vi "JTAG Base Function.vi"(0 "Function":u16(ring) items=["READ_IO_VARS"=0, "PORT_OUT"=1, "PORT_SEL"=2, "PORT_REN"=3, "PORT_IN"=4, "PORT_DIR"=5, "SET_LCM"=6, "PWR_WRITE_SINGLE"=12, "PWR_READ_SINGLE"=13, "PWR_WRITE_MASK"=16, "PWR_WRITE_TRIM_DEFAULTS"=17, "STIM_POWER_UP"=20, "STIM_POWER_DN"=21, "STIM_WRITE_SINGLE"=22, "STIM_READ_SINGLE"=23, "STIM_WRITE_BLOCK"=24, "STIM_READ_BLOCK"=25, "STIM_WRITE_MASK"=26, "MICS_POWER_UP"=30, "MICS_WAKEUP_PULSE"=205, "MICS_POWER_DN"=31, "MICS_WRITE_SINGLE"=32, "MICS_READ_SINGLE"=33, "MICS_WRITE_BLOCK"=34, "MICS_READ_BLOCK"=35, "MICS_WRITE_MASK"=36, "MEM_POWER_UP"=40, "MEM_POWER_DN"=41, "MEM_WRITE_SINGLE"=42, "MEM_READ_SINGLE"=43, "MEM_WRITE_BLOCK"=44, "MEM_READ_BLOCK"=45, "MEM_WRITE_MASK"=46, "MEM_WRITE_SR"=47, "MEM_READ_SR"=48, "MEM_WRITE_OPCODE"=49, "INIT_PORTS"=50, "INIT_COMMS"=60, "RELEASE_COMMS"=61, "INIT_VARS"=62, "DCO_1MHZ"=63, "DCO_8MHZ"=64, "STANDARD_STARTUP"=65, "SET_LCM"=66, "PLUTO_WRITE_TRIM_DEFAULTS"=67, "SATURN_DIG_STARTUP"=68, "SATURN_BBC_STARTUP"=69, "SATURN_BBC_SHUTDOWN"=70, "SATURN_AUTO_FULL_STARTUP"=71, "SATURN_FULL_SHUTDOWN"=72, "SATURN_ENABLE_PROGRAMMING"=73, "SATURN_ENABLE_SEQUENCER"=74, "START_STIM_CLK"=80, "STOP_STIM_CLK"=81, "PULSE_STIM_CLK"=82, "PULSE_STIM_SCK"=83, "SINGLE_ADC12"=85, "SINGLE_ADC12_REPEAT"=86, "MULTI_ADC12"=87, "MULTI_ADC12_REPEAT"=88, "DISABLE_ADC12"=89, "READ_CLOCK_REGISTERS"=90, "WRITE_CLOCK_REGISTERS"=91, "TC_STIM_RAM_READ"=200, "TC_STIM_RAM_WRITE"=201, "TC_STIM_PHASE_REGS_READ"=202, "TC_STIM_PHASE_REGS_WRITE"=203, "TC_BROWN_OUT_TEST"=204, "TC_TIMING_TEST"=220], 1 "ARG 4":u16 format="%04x", 2 "ARG 5":u16 format="%04x", 3 "ARG 6":u16 format="%04x", 5 "ARG 1":u16 format="%04x", 7 "ARG 2":u16 format="%04x", 9 "ARG 3":u16 format="%04x", 11 "error in (no error)":errorcluster) -> (4 "ARG 7":u16 format="%04x", 8 "ARG1-ARG7":u16[](array[numeric]) format="%04x", 15 "error out":errorcluster)   [LabVIEW 2010]
panel:
  # "ARG1"
  # "ARG2"
  # "ARG3"
  # "ARG4"
  # "ARG5"
  # "ARG6"
  # "ARG7"
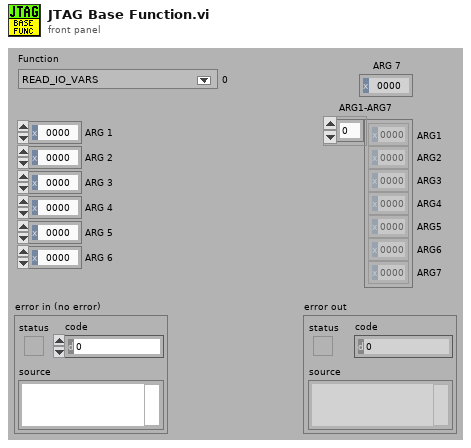
[diagram p1: front panel]
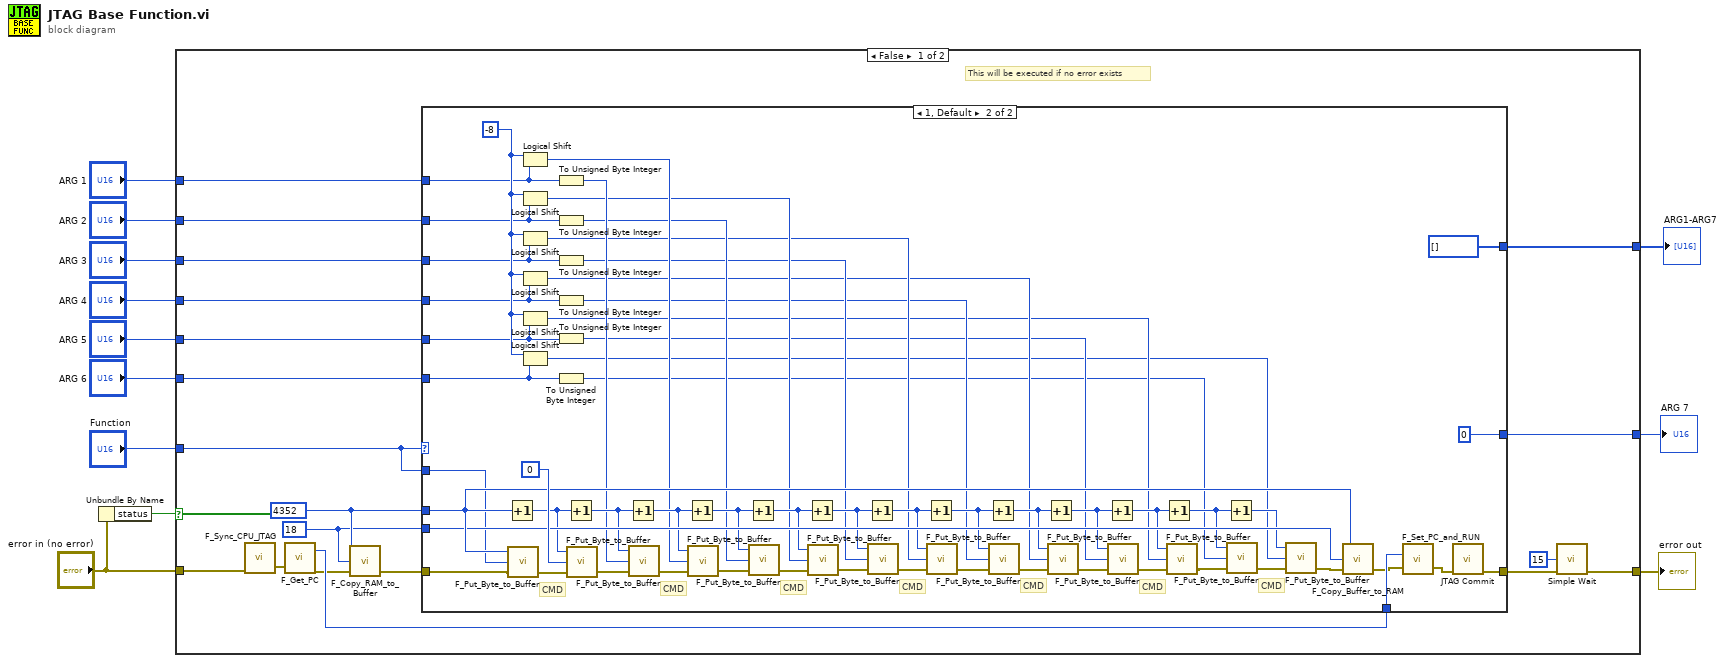
[diagram p0: block diagram]
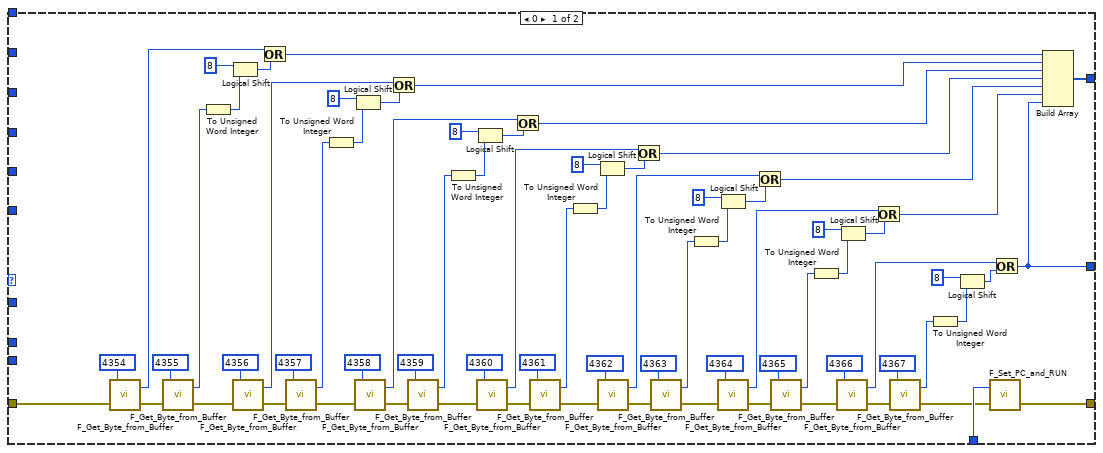
[diagram p2: hidden frame]
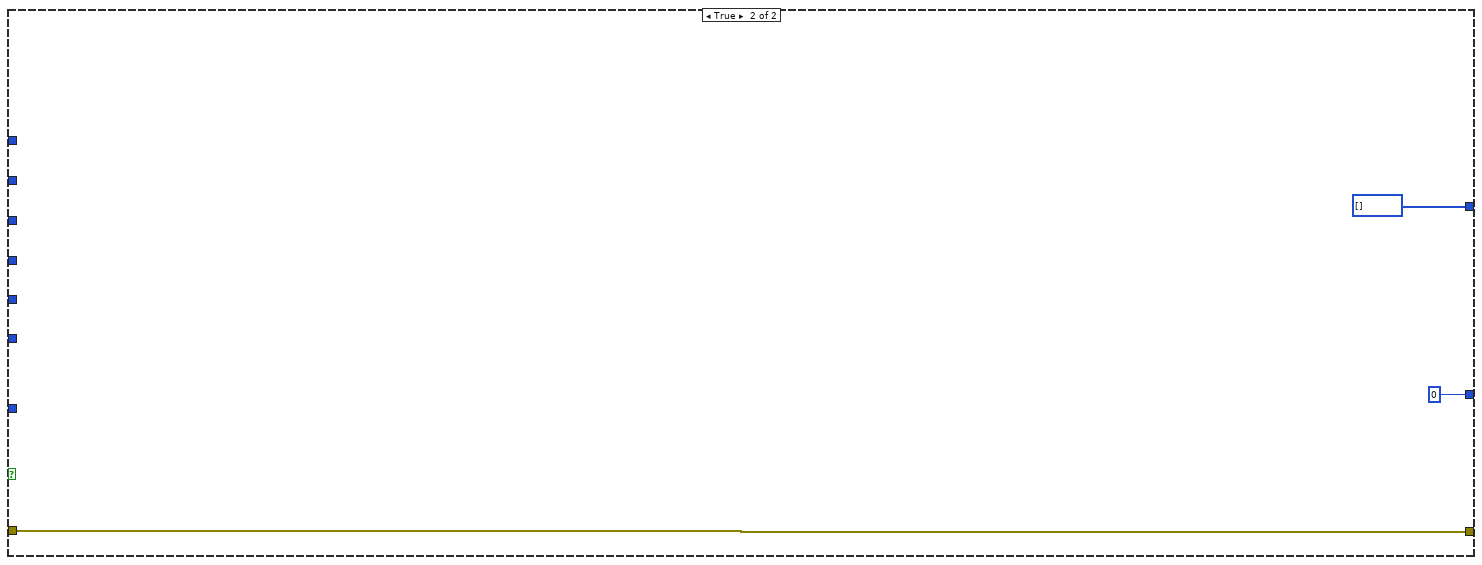
[diagram p3: hidden frame]
diagram:
  n1 = Unbundle By Name("error in (no error)") -> ("status"=w11:bool)
  n2 = case shown="False" w11 {
    tunnel: [w16 w165] -> w12
    tunnel: "error in (no error)" -> [w31 w165]
    tunnel: "Function" -> [w13 _]
    tunnel: "ARG 6" -> [w20 _]
    tunnel: "ARG 5" -> [w21 _]
    tunnel: "ARG 4" -> [w22 _]
    tunnel: "ARG 3" -> [w23 _]
    tunnel: "ARG 2" -> [w24 _]
    tunnel: "ARG 1" -> [w25 _]
    tunnel: [w15 u16 0 ("ARG 7")] -> w3
    tunnel: [w14 u16[] []] -> w2
    frame False {
      w29 = u16 18
      w30 = u16 4352
      # "This will be executed if no error exists"
      n3 = call "F_Sync_CPU_JTAG.vi"("error in (no error)"=w31) -> ("error out"=w27:errorcluster)  [unwired: 1 in, 1 out]
      n4 = call "F_Get_PC.vi"("error in (no error)"=w27) -> ("error out"=w19:errorcluster, "Program Counter"=w26:u16)  [unwired: 1 in]
      n5 = call "F_Copy_RAM_to_Buffer.vi"("error in (no error)"=w19, "Block size to be copied"=w29, "RAM start address"=w30) -> ("error out"=w28:errorcluster)  [unwired: 2 in]
      n6 = case shown="1, Default" w13 {
        tunnel: w30 -> [_ w160]
        tunnel: w29 -> [_ w159]
        tunnel: w28 -> [w58 w158]
        tunnel: w13 -> [_ w157]
        tunnel: w26 -> [w105 w156]
        tunnel: w25 -> [_ w128]
        tunnel: w24 -> [_ w127]
        tunnel: w23 -> [_ w126]
        tunnel: w22 -> [_ w125]
        tunnel: w21 -> [_ w124]
        tunnel: w20 -> [_ w123]
        tunnel: [w104 w108] -> w17
        tunnel: [w51 u16 0 ("ARG 7")] -> w15
        tunnel: [w32 u16[] []] -> w14
        frame 0 {
          n7 = call "F_Get_Byte_from_Buffer.vi"("error in (no error)"=w58, "Address of byte to be read"=u16 4354) -> ("error out"=w64:errorcluster, "Current value"=w44:u8)
          n8 = call "F_Get_Byte_from_Buffer.vi"("error in (no error)"=w64, "Address of byte to be read"=u16 4355) -> ("error out"=w52:errorcluster, "Current value"=w60:u8)
          n9 = To Unsigned Word Integer(number=w60) -> (unsigned 16bit integer=w59:u16)
          n10 = Logical Shift(y=i16 8, x=w59) -> (x << y=w50:u16)
          n11 = call "F_Get_Byte_from_Buffer.vi"("error in (no error)"=w52, "Address of byte to be read"=u16 4356) -> ("error out"=w70:errorcluster, "Current value"=w43:u8)
          n12 = Or(x=w44, y=w50) -> (x .or. y?=w33:u16)
          n13 = call "F_Get_Byte_from_Buffer.vi"("error in (no error)"=w70, "Address of byte to be read"=u16 4357) -> ("error out"=w53:errorcluster, "Current value"=w66:u8)
          n14 = To Unsigned Word Integer(number=w66) -> (unsigned 16bit integer=w65:u16)
          n15 = Logical Shift(y=i16 8, x=w65) -> (x << y=w49:u16)
          n16 = call "F_Get_Byte_from_Buffer.vi"("error in (no error)"=w53, "Address of byte to be read"=u16 4358) -> ("error out"=w76:errorcluster, "Current value"=w42:u8)
          n17 = Or(x=w43, y=w49) -> (x .or. y?=w34:u16)
          n18 = call "F_Get_Byte_from_Buffer.vi"("error in (no error)"=w76, "Address of byte to be read"=u16 4359) -> ("error out"=w54:errorcluster, "Current value"=w72:u8)
          n19 = To Unsigned Word Integer(number=w72) -> (unsigned 16bit integer=w71:u16)
          n20 = Logical Shift(y=i16 8, x=w71) -> (x << y=w48:u16)
          n21 = call "F_Get_Byte_from_Buffer.vi"("error in (no error)"=w54, "Address of byte to be read"=u16 4360) -> ("error out"=w82:errorcluster, "Current value"=w41:u8)
          n22 = Or(x=w42, y=w48) -> (x .or. y?=w35:u16)
          n23 = call "F_Get_Byte_from_Buffer.vi"("error in (no error)"=w82, "Address of byte to be read"=u16 4361) -> ("error out"=w55:errorcluster, "Current value"=w78:u8)
          n24 = To Unsigned Word Integer(number=w78) -> (unsigned 16bit integer=w77:u16)
          n25 = Logical Shift(y=i16 8, x=w77) -> (x << y=w47:u16)
          n26 = call "F_Get_Byte_from_Buffer.vi"("error in (no error)"=w55, "Address of byte to be read"=u16 4362) -> ("error out"=w88:errorcluster, "Current value"=w40:u8)
          n27 = Or(x=w41, y=w47) -> (x .or. y?=w36:u16)
          n28 = call "F_Get_Byte_from_Buffer.vi"("error in (no error)"=w88, "Address of byte to be read"=u16 4363) -> ("error out"=w56:errorcluster, "Current value"=w84:u8)
          n29 = To Unsigned Word Integer(number=w84) -> (unsigned 16bit integer=w83:u16)
          n30 = Logical Shift(y=i16 8, x=w83) -> (x << y=w46:u16)
          n31 = call "F_Get_Byte_from_Buffer.vi"("error in (no error)"=w56, "Address of byte to be read"=u16 4364) -> ("error out"=w94:errorcluster, "Current value"=w39:u8)
          n32 = Or(x=w40, y=w46) -> (x .or. y?=w37:u16)
          n33 = call "F_Get_Byte_from_Buffer.vi"("error in (no error)"=w94, "Address of byte to be read"=u16 4365) -> ("error out"=w57:errorcluster, "Current value"=w90:u8)
          n34 = To Unsigned Word Integer(number=w90) -> (unsigned 16bit integer=w89:u16)
          n35 = call "F_Get_Byte_from_Buffer.vi"("error in (no error)"=w57, "Address of byte to be read"=u16 4366) -> ("error out"=w103:errorcluster, "Current value"=w99:u8)
          n36 = Logical Shift(y=i16 8, x=w89) -> (x << y=w45:u16)
          n37 = Or(x=w39, y=w45) -> (x .or. y?=w38:u16)
          n38 = call "F_Get_Byte_from_Buffer.vi"("error in (no error)"=w103, "Address of byte to be read"=u16 4367) -> ("error out"=w102:errorcluster, "Current value"=w96:u8)
          n39 = To Unsigned Word Integer(number=w96) -> (unsigned 16bit integer=w95:u16)
          n40 = Logical Shift(y=i16 8, x=w95) -> (x << y=w97:u16)
          n41 = call "F_Set_PC_and_RUN.vi"("error in (no error)"=w102, "PC start address"=w105) -> ("error out"=w104:errorcluster)  [unwired: 1 in]
          n42 = Or(x=w99, y=w97) -> (x .or. y?=w51:u16)
          n43 = Build Array(w33, w34, w35, w36, w37, w38, w51) -> (w32:u16[])
        }
        frame 1, Default {
          w130 = -8
          # "CMD"
          # "CMD"
          # "CMD"
          # "CMD"
          # "CMD"
          # "CMD"
          # "CMD"
          n44 = Increment(x=w160) -> (x+1=w148:u16)
          n45 = call "F_Put_Byte_to_Buffer.vi"("error in (no error)"=w158, "New value"=w157, "Address of byte to be updated"=w160) -> ("error out"=w162:errorcluster)  [unwired: 2 in]
          n46 = Logical Shift(y=w130, x=w128) -> (x << y=w129:u16)
          n47 = Logical Shift(y=w130, x=w127) -> (x << y=w120:u16)
          n48 = Logical Shift(y=w130, x=w126) -> (x << y=w118:u16)
          n49 = Logical Shift(y=w130, x=w125) -> (x << y=w116:u16)
          n50 = Logical Shift(y=w130, x=w124) -> (x << y=w114:u16)
          n51 = Logical Shift(y=w130, x=w123) -> (x << y=w113:u16)
          n52 = To Unsigned Byte Integer(number=w128) -> (unsigned 8bit integer=w122:u8)
          n53 = To Unsigned Byte Integer(number=w127) -> (unsigned 8bit integer=w121:u8)
          n54 = To Unsigned Byte Integer(number=w126) -> (unsigned 8bit integer=w119:u8)
          n55 = To Unsigned Byte Integer(number=w125) -> (unsigned 8bit integer=w117:u8)
          n56 = To Unsigned Byte Integer(number=w124) -> (unsigned 8bit integer=w115:u8)
          n57 = To Unsigned Byte Integer(number=w123) -> (unsigned 8bit integer=w112:u8)
          n58 = Increment(x=w148) -> (x+1=w147:u16)
          n59 = call "F_Put_Byte_to_Buffer.vi"("error in (no error)"=w162, "New value"=u16 0, "Address of byte to be updated"=w148) -> ("error out"=w131:errorcluster)  [unwired: 2 in]
          n60 = Increment(x=w147) -> (x+1=w146:u16)
          n61 = call "F_Put_Byte_to_Buffer.vi"("error in (no error)"=w131, "New value"=w122, "Address of byte to be updated"=w147) -> ("error out"=w155:errorcluster)  [unwired: 2 in]
          n62 = Increment(x=w146) -> (x+1=w145:u16)
          n63 = call "F_Put_Byte_to_Buffer.vi"("error in (no error)"=w155, "New value"=w129, "Address of byte to be updated"=w146) -> ("error out"=w132:errorcluster)  [unwired: 2 in]
          n64 = Increment(x=w145) -> (x+1=w144:u16)
          n65 = call "F_Put_Byte_to_Buffer.vi"("error in (no error)"=w132, "New value"=w121, "Address of byte to be updated"=w145) -> ("error out"=w154:errorcluster)  [unwired: 2 in]
          n66 = Increment(x=w144) -> (x+1=w143:u16)
          n67 = call "F_Put_Byte_to_Buffer.vi"("error in (no error)"=w154, "New value"=w120, "Address of byte to be updated"=w144) -> ("error out"=w133:errorcluster)  [unwired: 2 in]
          n68 = Increment(x=w143) -> (x+1=w142:u16)
          n69 = call "F_Put_Byte_to_Buffer.vi"("error in (no error)"=w133, "New value"=w119, "Address of byte to be updated"=w143) -> ("error out"=w153:errorcluster)  [unwired: 2 in]
          n70 = Increment(x=w142) -> (x+1=w141:u16)
          n71 = call "F_Put_Byte_to_Buffer.vi"("error in (no error)"=w153, "New value"=w118, "Address of byte to be updated"=w142) -> ("error out"=w134:errorcluster)  [unwired: 2 in]
          n72 = Increment(x=w141) -> (x+1=w140:u16)
          n73 = call "F_Put_Byte_to_Buffer.vi"("error in (no error)"=w134, "New value"=w117, "Address of byte to be updated"=w141) -> ("error out"=w152:errorcluster)  [unwired: 2 in]
          n74 = Increment(x=w140) -> (x+1=w139:u16)
          n75 = call "F_Put_Byte_to_Buffer.vi"("error in (no error)"=w152, "New value"=w116, "Address of byte to be updated"=w140) -> ("error out"=w135:errorcluster)  [unwired: 2 in]
          n76 = Increment(x=w139) -> (x+1=w138:u16)
          n77 = call "F_Put_Byte_to_Buffer.vi"("error in (no error)"=w135, "New value"=w115, "Address of byte to be updated"=w139) -> ("error out"=w151:errorcluster)  [unwired: 2 in]
          n78 = Increment(x=w138) -> (x+1=w137:u16)
          n79 = call "F_Put_Byte_to_Buffer.vi"("error in (no error)"=w151, "New value"=w114, "Address of byte to be updated"=w138) -> ("error out"=w136:errorcluster)  [unwired: 2 in]
          n80 = Increment(x=w137) -> (x+1=w149:u16)
          n81 = call "F_Put_Byte_to_Buffer.vi"("error in (no error)"=w136, "New value"=w112, "Address of byte to be updated"=w137) -> ("error out"=w150:errorcluster)  [unwired: 2 in]
          n82 = call "F_Put_Byte_to_Buffer.vi"("error in (no error)"=w150, "New value"=w113, "Address of byte to be updated"=w149) -> ("error out"=w111:errorcluster)  [unwired: 2 in]
          n83 = call "F_Copy_Buffer_to_RAM.vi"("error in (no error)"=w111, "Block size to be copied"=w159, "Buffer start address"=w160) -> ("error out"=w110:errorcluster)  [unwired: 2 in]
          n84 = call "F_Set_PC_and_RUN.vi"("error in (no error)"=w110, "PC start address"=w156) -> ("error out"=w109:errorcluster)  [unwired: 1 in]
          n85 = call "JTAG Commit.vi"("error in (no error)"=w109) -> ("error out"=w108:errorcluster)  [unwired: 10 in]
        }
      }
      n86 = call "Simple Wait.vi"("mS"=u32 15, "error in"=w17) -> ("error out"=w16:errorcluster)  [unwired: 12 in, 1 out]
    }
    frame True {
      # "Error exists, skip all functions"
    }
  }
  "error out" <- w12
  "ARG 7" <- w3
  "ARG1-ARG7" <- w2
